vi "test_rt.vi"() -> ()   [LabVIEW 2014]
uses:
  <vilib>/addons/Control Design/_Model Construction/Model Typedefs.llb/CD State Space Model (MIMO).ctl
  <vilib>/addons/Control Design/_Model Construction/Model Typedefs.llb/CD General Elements.ctl
  <vilib>/FPGAPlugInAG/sbRIO-9632/niLvFpga_Open_sbRIO-9632.vi
  <vilib>/rvi/interface/common/dynamic/niFpgaDynamicAddResources.vi
  <vilib>/FPGAPlugInAG/Dynamic/niLvFpga_Reset_Dynamic.vi
  <vilib>/FPGAPlugInAG/Dynamic/niLvFpga_Run_Dynamic.vi
  <vilib>/Utility/error.llb/Error Cluster From Error Code.vi
  <vilib>/rvi/errors/niLvFpgaAdjustHostInterfaceError.vi
  <vilib>/FPGAPlugInAG/Dynamic/niLvFpga_Close_Dynamic.vi
  <vilib>/rvi/interface/nirviOpenFPGA/nirviOpenFPGA.xnode
  FPGA Bitfiles/PPDControlLab3fo_FPGATarget2_testfpga_kavfe-OOnFs.lvbitx
  <vilib>/rvi/interface/nirviMethod/nirviMethod.xnode
  <vilib>/rvi/interface/nirviReadWriteControl/nirviReadWriteControl.xnode
  <vilib>/rvi/interface/nirviCloseFPGA/nirviCloseFPGA.xnode
  <vilib>/rvi/interface/Simulation/niFpgaSimulationCallBeginRW.vi
  NiFpgaLv.dll
  <vilib>/addons/Control Design/_State Feedback Control/NI_CD_State Feedback Control.lvlib
  <vilib>/addons/Control Design/_Model Construction/NI_LinSys_Model Typedefs.lvlib
panel:
  out "Ang Vel":cluster{sgl[], sgl[]}(graph)
  out "velocity":cluster{sgl[], sgl[]}(graph)
  in  "da":sgl=3.0
  in  "a":sgl=13.0
  in  "dx":sgl=10.0
  in  "x":sgl=16.0
  out "Angle":cluster{sgl[], sgl[]}(graph)
  out "Pos":cluster{sgl[], sgl[]}(graph)
  out "Current":cluster{sgl[], dbl[]}(graph)
  out "Current Input":dbl=0.8923749923706055
  out "Angular Velocity":sgl=-1.5339805
  out "Velocity":sgl=0.33575112
  out "Gain":dbl[][](array[numeric])=[[13.022005449610596, 14.716197534981571, 47.807799727002596, 6.526245516742467]] format="%.2f"
  out "Angle":sgl=-0.021475721
  out "Position":sgl=0.0394525
  in  "Poles":cdb[](array[numeric])=[-1.9-10.0i, -1.9+10.0i, -1.6-1.3i, -1.6+1.3i] format="%.2f"
  in  "State-Space Model":T1={"properties"={"Model name"="", "Input names"=[], "Output names"=[], "Input Delays"=[], "Output Delays"=[], "Sampling Time"=0.002, "Notes"=""}, "A"=[[0.0, 1.0, 0.0, 0.0], [0.0, -6.81, -1.5, 0.0], [0.0, 0.0, 0.0, 1.0], [0.0, 15.4644, 25.658, 0.0]], "B"=[[0.0], [-1.52], [0.0], [3.4566]], "C"=[[1.0, 0.0, 0.0, 0.0], [0.0, 0.0, 1.0, 0.0]], "D"=[[0.0], [0.0]], "StateNames"=[], "Transport Delay"=[]} {"Transport Delay" format="%.2f"; "D" format="%#.2g"; "C" format="%#.2g"; "B" format="%#.2g"; "A" format="%#.2g"; "properties"."Sampling Time" format="%#.6p"; "properties"."Output Delays" format="%.4f"; "properties"."Input Delays" format="%.4f"}
  in  "stop":bool
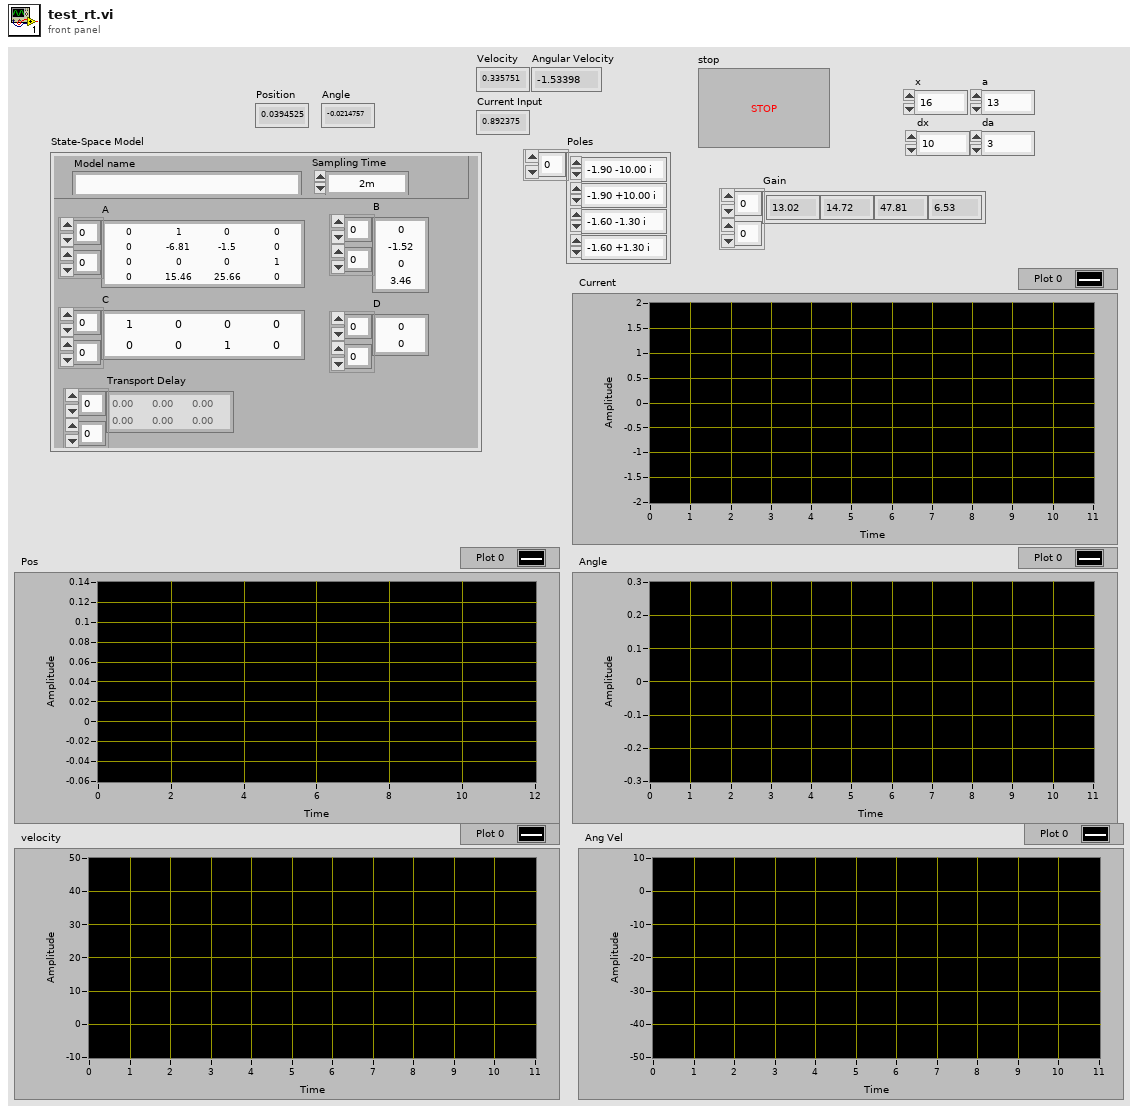
[diagram p1: front panel]
types:
  T1 = typedef "NI_LinSys_Model Typedefs.lvlib/CD State Space Model (MIMO).ctl" = cluster{"properties":T2, "A":dbl[][], "B":dbl[][], "C":dbl[][], "D":dbl[][], "StateNames":string[], "Transport Delay":dbl[][]}
  T2 = typedef "NI_LinSys_Model Typedefs.lvlib/CD General Elements.ctl" = cluster{"Model name":string, "Input names":string[], "Output names":string[], "Input Delays":dbl[], "Output Delays":dbl[], "Sampling Time":dbl, "Notes":string}
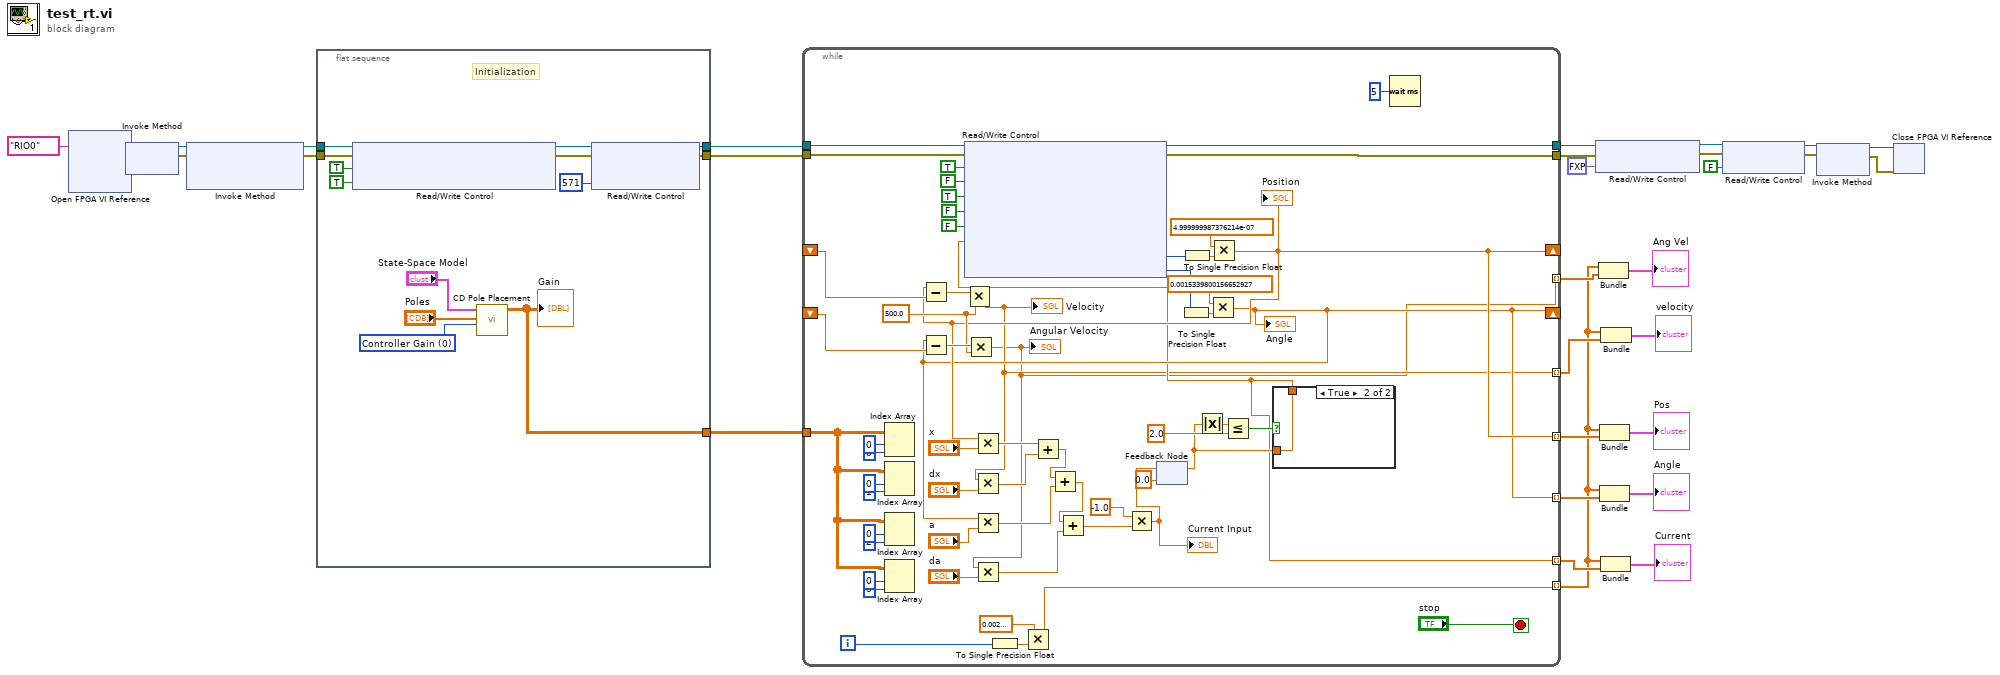
[diagram p0: block diagram]
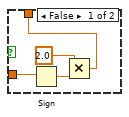
[diagram p2: hidden frame]
diagram:
  n1 = xnode "Open FPGA VI Reference"("resource name"=tag "RIO0") -> ("FPGA VI Reference Out"=w30:refnum<k20>, "error out"=w29:errorcluster)  [unwired: 1 in]
  n2 = xnode "Invoke Method"("FPGA VI Reference In"=w30, "error in"=w29) -> ("FPGA VI Reference Out"=w28:refnum<k20>, "error out"=w27:errorcluster)
  n3 = xnode "Invoke Method"("FPGA VI Reference In"=w28, "error in"=w27) -> ("FPGA VI Reference Out"=w26:refnum<k20>, "error out"=w25:errorcluster)  [unwired: 1 in]
  n4 = flat-sequence {
    tunnel: w26 -> [w44]
    tunnel: w25 -> [w43]
    tunnel: [w37] -> w24
    tunnel: [w36] -> w23
    tunnel: [w33] -> w12
    frame #0 {
      w32 = u16 0 items=["Controller Gain", "Observer Gain (Predictive)", "Observer Gain (Current)"] ("Gain Type")
      # "Initialization"
      n5 = xnode "Read/Write Control"("FPGA VI Reference In"=w44, "error in"=w43, "quad reset (Port0/DIO0,Port0/DIO1)"=TRUE, "Pendulum Reset"=TRUE) -> ("FPGA VI Reference Out"=w40:refnum<k20>, "error out"=w39:errorcluster)
      n6 = call <vilib>:"CD Pole Placement.vi"("Gain Type"=w32, "Poles"="Poles", "State-Space Model"="State-Space Model") -> ("Gain"=w33:dbl[][])  [unwired: 6 in, 2 out]
      "Gain" <- w33
      n7 = xnode "Read/Write Control"("FPGA VI Reference In"=w40, "error in"=w39, "Loop Rate (Ticks)"=u32 571) -> ("FPGA VI Reference Out"=w37:refnum<k20>, "error out"=w36:errorcluster)  [unwired: 1 in]
    }
  }
  n8 = while {
    tunnel: w24 -> [w102]
    tunnel: w23 -> [w101]
    tunnel: [w94] -> w17
    tunnel: [w93] -> w15
    tunnel: w12 -> [w72]
    shift-right: [w53] -> _
    shift-left: _ -> [w85]
    shift-right: [w52] -> _
    shift-left: _ -> [w84]
    tunnel: [w59] -> w2 mode=indexing
    tunnel: [w51] -> w11 mode=indexing
    tunnel: [w53] -> w9 mode=indexing
    tunnel: [w52] -> w8 mode=indexing
    tunnel: [w46] -> w4 mode=indexing
    tunnel: [w45] -> w3 mode=indexing
    i -> [w62]
    stop <- "stop" stop-if-true
    w81 = sgl 500.0 ("y")
    n9 = Index Array(array=w72, index (row)=0, index (col)=0) -> ()  [unwired: 1 out]
    n10 = Index Array(array=w72, index (row)=0, index (col)=1) -> ()  [unwired: 1 out]
    n11 = Index Array(array=w72, index (row)=0, index (col)=2) -> ()  [unwired: 1 out]
    n12 = Index Array(array=w72, index (row)=0, index (col)=3) -> ()  [unwired: 1 out]
    n13 = To Single Precision Float(number=w62) -> (single precision float=w61:sgl)
    n14 = Multiply(x=sgl 0.002, y=w61) -> (x*y=w59:sgl)
    n15 = feedback #1(0.0) -> (w54:dbl)
    n16 = Absolute Value(x=w54) -> (abs(x)=w55:dbl)
    n17 = Less Or Equal?(x=w55, y=2.0) -> (x <= y?=w57:bool)
    n18 = case shown="True" w57 {
      tunnel: w54 -> [w106 w107]
      tunnel: [w103 w107] -> w51
      frame False {
        n19 = Sign(1:w106) -> (0:w105:dbl)
        n20 = Multiply(x=2.0, y=w105) -> (x*y=w103:dbl)
      }
      frame True {
      }
    }
    n21 = xnode "Read/Write Control"("FPGA VI Reference In"=w102, "error in"=w101, "Amp Enable"=TRUE, "Amp Reset"=FALSE, "Brake"=TRUE, "quad reset (Port0/DIO0,Port0/DIO1)"=FALSE, "Pendulum Reset"=FALSE, "Drive Command"=w51) -> ("FPGA VI Reference Out"=w94:refnum<k20>, "error out"=w93:errorcluster, "_quad pos (Port0/DIO0,Port0/DIO1)"=w90:i32, "Pendulum Position"=w87:i32)
    n22 = To Single Precision Float(number=w87) -> (single precision float=w88:sgl)
    n23 = To Single Precision Float(number=w90) -> (single precision float=w91:sgl)
    n24 = Multiply(x=sgl 0.00153398, y=w88) -> (x*y=w52:sgl)
    "Angle" <- w52
    n25 = Subtract(x=w52, y=w84) -> (x-y=w82:sgl)
    n26 = Multiply(x=w82, y=w81) -> (x*y=w45:sgl)
    "Angular Velocity" <- w45
    n27 = Multiply(x=w52, y="a") -> (x*y=w68:sgl)
    n28 = Multiply(x=w45, y="da") -> (x*y=w66:sgl)
    n29 = Multiply(x=sgl 5e-07, y=w91) -> (x*y=w53:sgl)
    "Position" <- w53
    n30 = Subtract(x=w53, y=w85) -> (x-y=w83:sgl)
    n31 = Multiply(x=w83, y=w81) -> (x*y=w46:sgl)
    "Velocity" <- w46
    n32 = Multiply(x=w53, y="x") -> (x*y=w71:sgl)
    n33 = Multiply(x=w46, y="dx") -> (x*y=w70:sgl)
    n34 = Add(x=w71, y=w70) -> (x+y=w69:sgl)
    n35 = Add(x=w69, y=w68) -> (x+y=w67:sgl)
    n36 = Add(x=w67, y=w66) -> (x+y=w65:sgl)
    n37 = Multiply(x=-1.0, y=w65) -> (x*y=w58:dbl)
    "Current Input" <- w58
    n38 = feedback-in #1(w58) -> ()
    n39 = Wait (ms)(milliseconds to wait=u32 5) -> ()  [unwired: 1 out]
  }
  n40 = xnode "Read/Write Control"("FPGA VI Reference In"=w17, "error in"=w15, "Drive Command"=fxp<+/-,20,5> 0.0) -> ("FPGA VI Reference Out"=w16:refnum<k20>, "error out"=w14:errorcluster)
  n41 = Bundle(w2, w3) -> (→"Ang Vel":cluster{sgl[], sgl[]})  [unwired: 1 in]
  n42 = Bundle(w2, w9) -> (→"Pos":cluster{sgl[], sgl[]})  [unwired: 1 in]
  n43 = Bundle(w2, w8) -> (→"Angle":cluster{sgl[], sgl[]})  [unwired: 1 in]
  n44 = Bundle(w2, w11) -> (→"Current":cluster{sgl[], dbl[]})  [unwired: 1 in]
  n45 = Bundle(w2, w4) -> (→"velocity":cluster{sgl[], sgl[]})  [unwired: 1 in]
  n46 = xnode "Read/Write Control"("FPGA VI Reference In"=w16, "error in"=w14, "Amp Enable"=FALSE) -> ("FPGA VI Reference Out"=w20:refnum<k20>, "error out"=w19:errorcluster)
  n47 = xnode "Invoke Method"("FPGA VI Reference In"=w20, "error in"=w19) -> ("FPGA VI Reference Out"=w22:refnum<k20>, "error out"=w21:errorcluster)
  n48 = xnode "Close FPGA VI Reference"("FPGA VI Reference In"=w22, "error in"=w21) -> ()  [unwired: 1 out]
